vi "Dynamic_call_global.ph.vi"() -> ()   [LabVIEW 2010]
panel:
  in  "Take LDA PWA & An":refnum<vi>
  in  "Initial Plug Ins Extra":string[](array[string])
  in  "Per Block Plug Ins Extra":string[](array[string])
  in  "GPIB_Server.vi":refnum<vi>
  out "EnFlo Hub running?":bool
  in  "Final Plug Ins":string[](array[string])
  in  "Per Block Plug Ins":string[](array[string])
  in  "Initial Plug Ins":string[](array[string])
  in  "Acquisition Interlock":bool
  in  "Error Cluster":errorcluster
  in  "Client Name":string
  in  "Scanning Valve Driver":refnum<vi>
  in  "Program Active server":refnum<vi>
  in  "Ready to take data?":T1
  in  "Take data":refnum<k4>
  in  "Opened VIs":string[](array[string])
  in  "Plug in":refnum<vi>
  in  "Analogue Input":refnum<vi>
  in  "Plug in values":string[](array[string])
  in  "Plug in titles":string[](array[string])
  in  "Remote Subvi Opened":refnum<k4>
  in  "VI name to launch":string
  in  "Call Remote Subvi":refnum<k4>
  # "These Globals are used to enable the time to commence\nData acquistion to be controlled by code running in parallel\nwith the measurement program if Interlock is true."
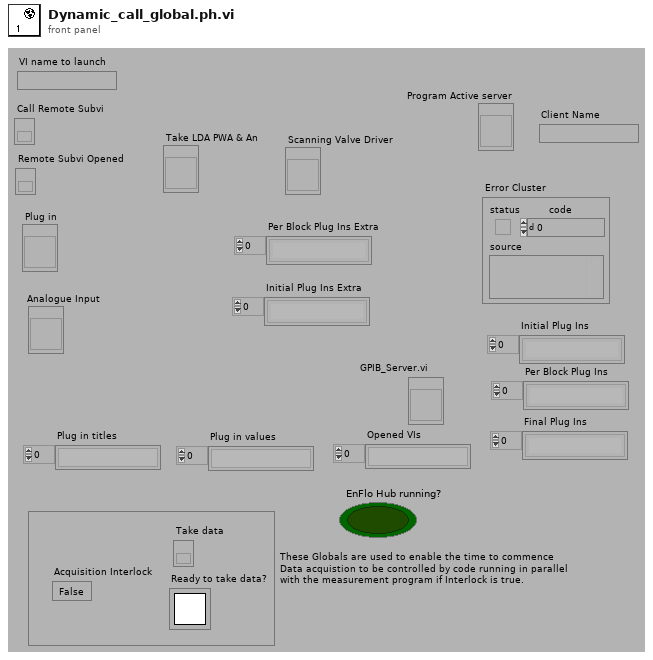
[diagram p1: front panel]
types:
  T1 = typedef "Rendezvous RefNum" = refnum<k1>
diagram:
